vi "Set Codes on all Error Channels.vi"(8 "error in (no error)":errorcluster, 10 "Error Codes":cluster{"Code":i32, "String":string}[](array[cluster]), 11 "Node Ptr in":u64) -> (0 "error out":errorcluster, 3 "Section Ref out":T1 format="%.0x")   [LabVIEW 2018, in "Instrument Addon Shared.lvlib"]
uses:
  Instrument Addon Shared.lvlib
  Constants.vi
  <vilib>/NI/NI VeriStand Advanced SysDef API/SysDef API/Advanced System Definition.lvlib
  <vilib>/NI/NI VeriStand Advanced SysDef API/_SubVIs/SysDef.Search.GUIDs.vi
  <vilib>/NI VeriStand/Custom Device API/Custom Device Item Ref.ctl
  <vilib>/NI VeriStand/Custom Device API/Custom Device API.lvlib
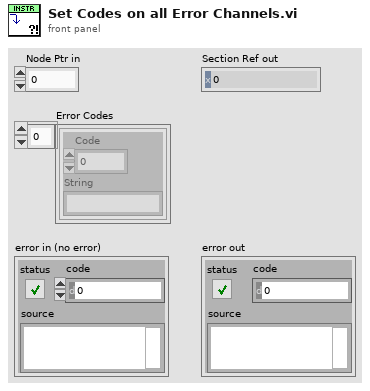
[diagram p1: front panel]
types:
  T1 = typedef "Custom Device API.lvlib/Custom Device Item Ref.ctl" = u64
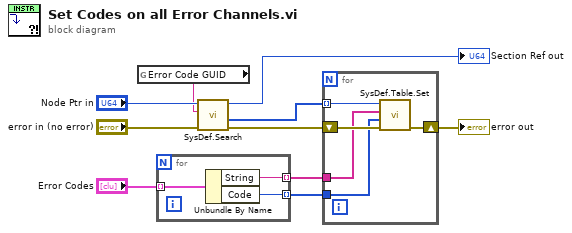
[diagram p0: block diagram]
diagram:
  n1 = global read "Constants.vi" "Error Code GUID"() -> (w1:string)
  n2 = for {
    tunnel: "Error Codes" -> [w13] mode=indexing
    tunnel: [w12] -> w4 mode=indexing
    tunnel: [w11] -> w5 mode=indexing
    n3 = Unbundle By Name(w13) -> ("String"=w12:string, "Code"=w11:i32)
  }
  n4 = call-poly <vilib>:"SysDef.Search.vi"("error in (no error)"="error in (no error)", "GUID"=w1, "nodeID"="Node Ptr in") -> ("error out"=w3:errorcluster, "Values Out"=w2:u64[], "nodeID out"=→"Section Ref out":u64)  [unwired: 5 in, 1 out]
  n5 = for {
    tunnel: w2 -> [w18] mode=indexing
    shift-right: [w16] -> w6
    shift-left: w3 -> [w17]
    tunnel: w4 -> [w15]
    tunnel: w5 -> [w14]
    n6 = call <vilib>:"SysDef.Table.Set.vi"("error in (no error)"=w17, "Values"=w14, "Names"=w15, "nodeID"=w18) -> ("error out"=w16:errorcluster)  [unwired: 6 in, 1 out]
  }
  "error out" <- w6
